vi "STICK_get_ports.vi"(5 "error in (no error)":errorcluster, 6 "VISA Refnum in":refnum<visa-resource-name>) -> (0 "error out":errorcluster, 1 "VISA Refnum out":refnum<visa-resource-name>, 2 "P2":T1, 3 "P1":T2, 4 "data":u8)   [LabVIEW 2014]
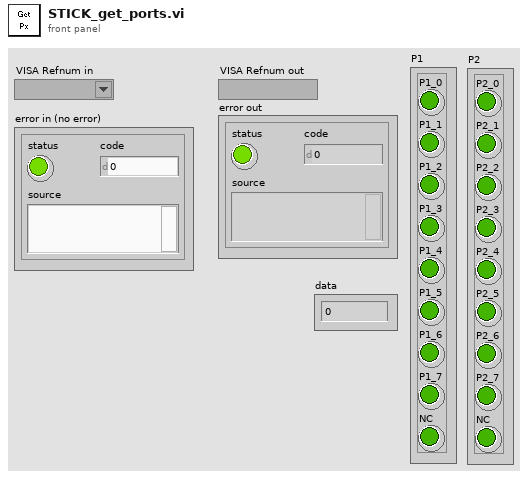
[diagram p1: front panel]
types:
  T1 = cluster{"P2_0":bool, "P2_1":bool, "P2_2":bool, "P2_3":bool, "P2_4":bool, "P2_5":bool, "P2_6":bool, "P2_7":bool, "NC":bool}
  T2 = cluster{"P1_0":bool, "P1_1":bool, "P1_2":bool, "P1_3":bool, "P1_4":bool, "P1_5":bool, "P1_6":bool, "P1_7":bool, "NC":bool}
  T3 = cluster{"Boolean array[0]":bool, "Boolean array[1]":bool, "Boolean array[2]":bool, "Boolean array[3]":bool, "Boolean array[4]":bool, "Boolean array[5]":bool, "Boolean array[6]":bool, "Boolean array[7]":bool, "Boolean array[8]":bool}
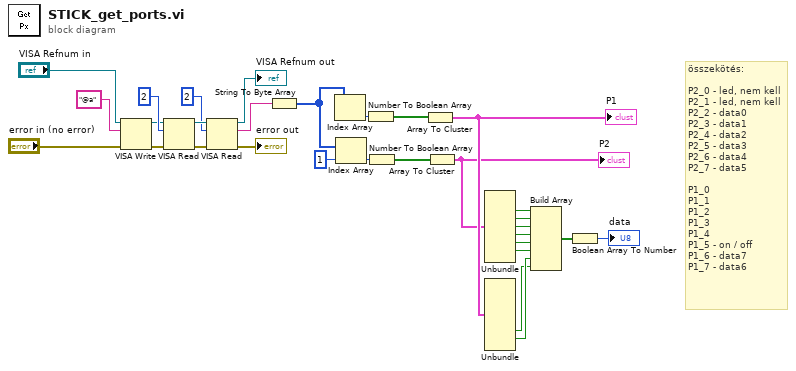
[diagram p0: block diagram]
diagram:
  # "összekötés: \n\nP2_0 - led, nem kell\nP2_1 - led, nem kell\nP2_2 - data0\nP2_3 - data1\nP2_4 - data2\nP2_5 - data3\nP2_6 - data4\nP2_7 - data5\n\nP1_0 \nP1_1\nP1_2\nP1_3\nP1_4\nP1_5 - on / off\nP1_6 - data7\nP1_7 - data6"
  n1 = VISA Write(VISA resource name="VISA Refnum in", write buffer="@a", error in (no error)="error in (no error)") -> (VISA resource name out=w27:refnum<visa-resource-name>, error out=w28:errorcluster)  [unwired: 1 out]
  n2 = VISA Read(VISA resource name=w27, byte count=u32 2, error in (no error)=w28) -> (VISA resource name out=w20:refnum<visa-resource-name>, error out=w21:errorcluster)  [unwired: 2 out]
  n3 = VISA Read(VISA resource name=w20, byte count=u32 2, error in (no error)=w21) -> (VISA resource name out=→"VISA Refnum out":refnum<visa-resource-name>, read buffer=w24:string, error out=→"error out":errorcluster)  [unwired: 1 out]
  n4 = String To Byte Array(string=w24) -> (unsigned byte array=w16:u8[])
  n5 = Index Array(array=w16) -> (element=w18:u8)  [unwired: 1 in]
  n6 = Index Array(array=w16, index=1) -> (element=w17:u8)
  n7 = Number To Boolean Array(number=w18) -> (Boolean array=w1:bool[])
  n8 = Number To Boolean Array(number=w17) -> (Boolean array=w2:bool[])
  n9 = Array To Cluster(array=w1) -> (cluster=w13:T3)
  "P1" <- w13
  n10 = Array To Cluster(array=w2) -> (cluster=w12:T3)
  "P2" <- w12
  n11 = Unbundle(w12) -> ("Boolean array[2]"=w11:bool, "Boolean array[3]"=w10:bool, "Boolean array[4]"=w9:bool, "Boolean array[5]"=w8:bool, "Boolean array[6]"=w7:bool, "Boolean array[7]"=w6:bool)  [unwired: 3 out]
  n12 = Unbundle(w13) -> ("Boolean array[6]"=w3:bool, "Boolean array[7]"=w4:bool)  [unwired: 7 out]
  n13 = Build Array(w11, w10, w9, w8, w7, w6, w4, w3) -> (w5:bool[])
  n14 = Boolean Array To Number(Boolean array=w5) -> (number=→"data":u32)
